vi "Cleanup.vi"(8 "error in (no error)":errorcluster, 11 "HAL Manager in":refnum<class "HAL Manager.lvclass">) -> (0 "error out":errorcluster)   [LabVIEW 2020, in "HAL.lvlib" / "HAL Manager.lvclass"]
uses:
  HAL Manager.lvclass
  HAL Manager.lvclass/HAL Manager.ctl
  Device/Device.lvclass
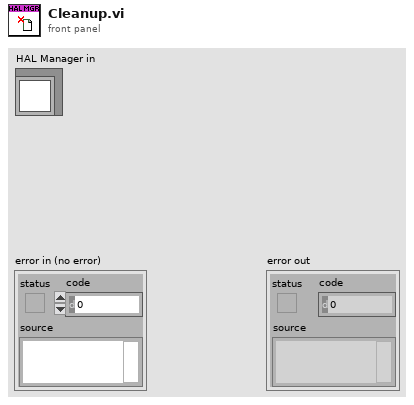
[diagram p1: front panel]
types:
  T1 = typedef "HAL.lvlib/HAL Manager.lvclass/Ref Data.ctl" = cluster{"Devices":refnum<class "Device.lvclass">[], "Type":string[], "Models":string[], "Name":string[]}
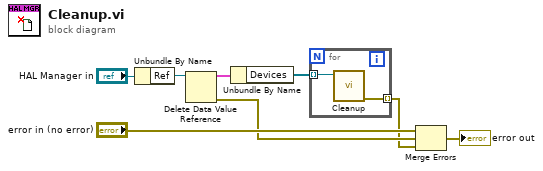
[diagram p0: block diagram]
diagram:
  n1 = Unbundle By Name("HAL Manager in") -> ("Ref"=w6:refnum<data-value>)
  n2 = Delete Data Value Reference(data value reference=w6) -> (data value=w5:T1, error out=w2:errorcluster)  [unwired: 1 in]
  n3 = Unbundle By Name(w5) -> ("Devices"=w4:refnum<class "Device.lvclass">[])
  n4 = for {
    tunnel: w4 -> [w10] mode=indexing
    tunnel: [w9] -> w1 mode=indexing
    n5 = call "Cleanup.vi"("Device in"=w10) -> ("error out"=w9:errorcluster)  [unwired: 10 in]
  }
  n6 = Merge Errors("error in (no error)", w2, w1) -> (→"error out":errorcluster)
